vi "Prototype.vi"(8 "error in (no error)":errorcluster, 10 "Reference Method Prototyper in":refnum<class "Reference Method Prototyper.lvclass">, 11 "Scripter in":refnum<class "Message Scripter.lvclass">) -> (0 "error out":errorcluster, 2 "Reference Method Prototyper out":refnum<class "Reference Method Prototyper.lvclass">, 3 "Scripter out":refnum<class "Message Scripter.lvclass">)   [LabVIEW 2020, in "Message Maker.lvlib" / "Reference Method Prototyper.lvclass"]
uses:
  Reference Method Prototyper.lvclass
  Message Maker.lvlib
  Message Scripter/Message Scripter.lvclass
  Abstract Icon Prototyper/Abstract Icon Prototyper.lvclass
  Prototyper/Prototyper.lvclass
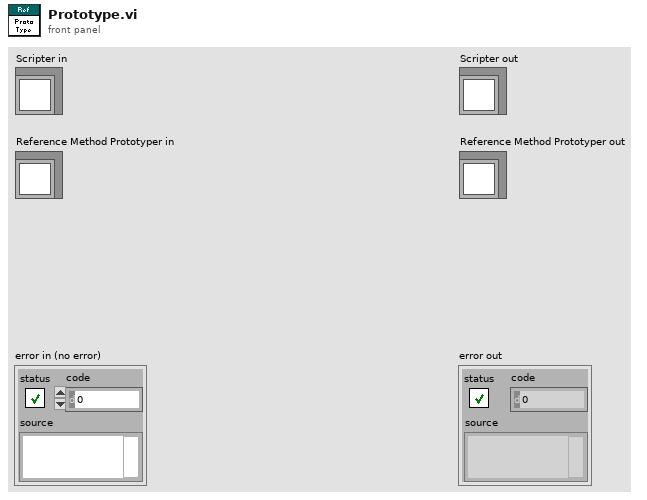
[diagram p1: front panel]
types:
  T1 = enum16{"Invalid Wire Rule", "Required", "Recommended", "Optional", "Dynamic Dispatch"}[]
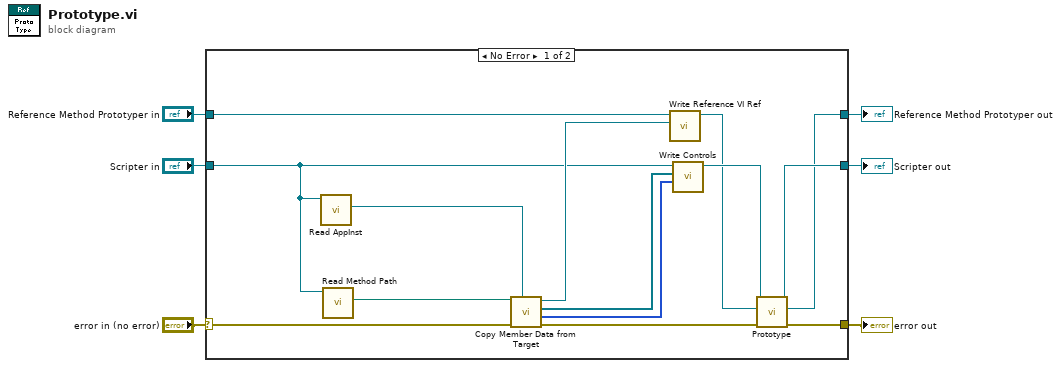
[diagram p0: block diagram]
diagram:
  n1 = case shown="No Error" "error in (no error)" {
    selector: "error in (no error)" -> [w18 w22]
    tunnel: "Scripter in" -> [w8 w23]
    tunnel: [w15 w23] -> w5
    tunnel: [w17 w22] -> w3
    tunnel: "Reference Method Prototyper in" -> [w11 w21]
    tunnel: [w14 w21] -> w1
    frame No Error {
      n2 = call "Read AppInst.vi"("Message Maker in"=w8) -> ("AppInst"=w19:refnum<vi>)  [unwired: 10 in]
      n3 = call "Read Method Path.vi"("Message Maker in"=w8) -> ("Method Path"=w7:path)  [unwired: 10 in]
      n4 = call "Copy Member Data from Target.vi"("AppInst"=w19, "error in (no error)"=w18, "Target Method path"=w7) -> ("error out"=w13:errorcluster, "Wiring Rules"=w12:T1, "Controls[]"=w20:refnum<vi>[], "Target Method Ref"=w9:refnum<vi>)  [unwired: 5 in]
      n5 = call "Write Reference VI Ref.vi"("Reference VI Ref"=w9, "Prototyper in"=w11) -> ("Prototyper out"=w10:refnum<class "Reference Method Prototyper.lvclass">)  [unwired: 9 in]
      n6 = call "Write Controls.vi"("Wiring Rules"=w12, "Controls[]"=w20, "Message Scripter in"=w8) -> ("Message Scripter out"=w16:refnum<class "Message Scripter.lvclass">)  [unwired: 8 in]
      n7 = call-parent "Prototype.vi"("error in (no error)"=w13, "Abstract Prototyper in"=w10, "Scripter in"=w16) -> ("error out"=w17:errorcluster, "Abstract Prototyper out"=w14:refnum<class "Reference Method Prototyper.lvclass">, "Scripter out"=w15:refnum<class "Message Scripter.lvclass">)  [unwired: 6 in]
    }
    frame Error {
    }
  }
  "error out" <- w3
  "Reference Method Prototyper out" <- w1
  "Scripter out" <- w5
